vi "main.vi"(8 "error in":errorcluster) -> (0 "error out":errorcluster)   [LabVIEW 2018, in "Controller.lvlib"]
uses:
  Controller.lvlib
  Common/Common.lvlib
  Common/vi/Stop All - Action.ctl
  ctl/Queue Actions.ctl
  ctl/Module State.ctl
  Error Handler/Error Handler/ctl/Module State.ctl
  Error Handler/Error Handler/Error Handler.lvlib
  Entry Console/Entry Console.lvlib
  Wash Display Console/Wash Display Console.lvlib
  Vehicle Position Interface/Vehicle Position Interface.lvlib
  Vehicle Position Interface/ctl/Module State.ctl
  Wash Display Console/ctl/Module State.ctl
  Entry Console/ctl/Module State.ctl
  ctl/Database Action.ctl
  Entry Console/ctl/Wash Step Selection Buttons.ctl
  Common/ctl/Wash Step.ctl
  Common/ctl/Station.ctl
  ctl/Database Record.ctl
  ctl/Countdown Timer Action.ctl
  Vehicle Position Interface/ctl/Vehicle Position.ctl
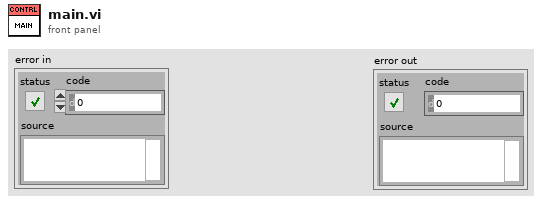
[diagram p1: front panel]
types:
  T1 = typedef "Entry Console.lvlib/Wash Step Selection Buttons.ctl" = cluster{"Under Body Wash":bool, "Bug Remover":bool, "Pre-Soak":bool, "High Pressure Wash (default)":bool, "Low Pressure Wax":bool, "Spot Free Rinse":bool, "Tire Shine Foam":bool, "Air Dry":bool}
  T2 = typedef "Common.lvlib/Wash Step.ctl" = enum16{"None", "Under Body Wash", "Bug Remover", "Pre-Soak", "High Pressure Wash (default)", "Low Pressure Wax", "Spot Free Rinse", "Tire Shine Foam", "Air Dry"}
  T3 = cluster{"Wash Steps Selected":T1, "Current Wash Step":T2, "Current State":enum16{"Wait", "Start", "Wait for vehicle Position", "Wash Step Execution", "Wash step/cycle completion", "Wash Step exit"}}
  T4 = typedef "Controller.lvlib/Module State.ctl" = enum16{"Init", "Idle", "Error", "Close", "Wait for Start State", "Start State", "Wait For Vehicle Position", "Wash Step Execution", "Wash Step/Cycle Completion", "Wash Exit State", "Wash Abort/Terminate State", "Entry Console: Start button pressed", "Entry Console: Wash Steps buttons Pressed", "Vehicle Position: Slider Moved", "Check Timer"}
  T5 = typedef "Controller.lvlib/Queue Actions.ctl" = enum16{"Create", "Get", "Destroy"}
  T6 = typedef "Common.lvlib/Stop All - Action.ctl" = enum16{"Create", "Get", "Fire", "Destroy"}
  T7 = typedef "Entry Console.lvlib/Module State.ctl" = enum16{"Init", "Idle", "Error", "Close", "Wash Step Selection Buttons: Enable/Disable All", "Wash Step Selection Buttons: Set All", "Wash Step Selection Buttons: Set Single (On/Off)", "Start: Enable/Disable", "Start: Set State (On/Off)"}
  T8 = typedef "Wash Display Console.lvlib/Module State.ctl" = enum16{"Init", "Idle", "Error", "Close", "Car Wash Indicators: Set All", "Car Wash Indicators: Set Single (On/Off)", "Wash Entry: Set State", "Vehicle Out of Position: Green/Red", "Time Remaining: Set"}
  T9 = typedef "Vehicle Position Interface.lvlib/Module State.ctl" = enum16{"Init", "Idle", "Error", "Close", "Vehicle Position: Set", "Vehicle Position: Send to controller"}
  T10 = typedef "Controller.lvlib/Database Action.ctl" = enum16{"Read Records (init)", "Get", "Query Timing Data", "Insert New Data record", "Update Data Record"}
  T11 = typedef "Error Handler.lvlib/Module State.ctl" = enum16{"Init", "Idle", "Error", "Close", "Handle External Error", "Log Error"}
  T12 = typedef "Controller.lvlib/Countdown Timer Action.ctl" = enum16{"Create (set goal time and start)", "Get (read)", "Reset"}
  T13 = typedef "Controller.lvlib/Database Record.ctl" = cluster{"Wash Step":T2, "Station":T14, "Wash Duration":dbl}
  T14 = typedef "Common.lvlib/Station.ctl" = enum16{"Entry", "Station 1", "Station 2", "Station 3", "Exit"}
  T15 = enum16{"Wait", "Start", "Wait for vehicle Position", "Wash Step Execution", "Wash step/cycle completion", "Wash Step exit"}
  T16 = typedef "Vehicle Position Interface.lvlib/Vehicle Position.ctl" = dbl
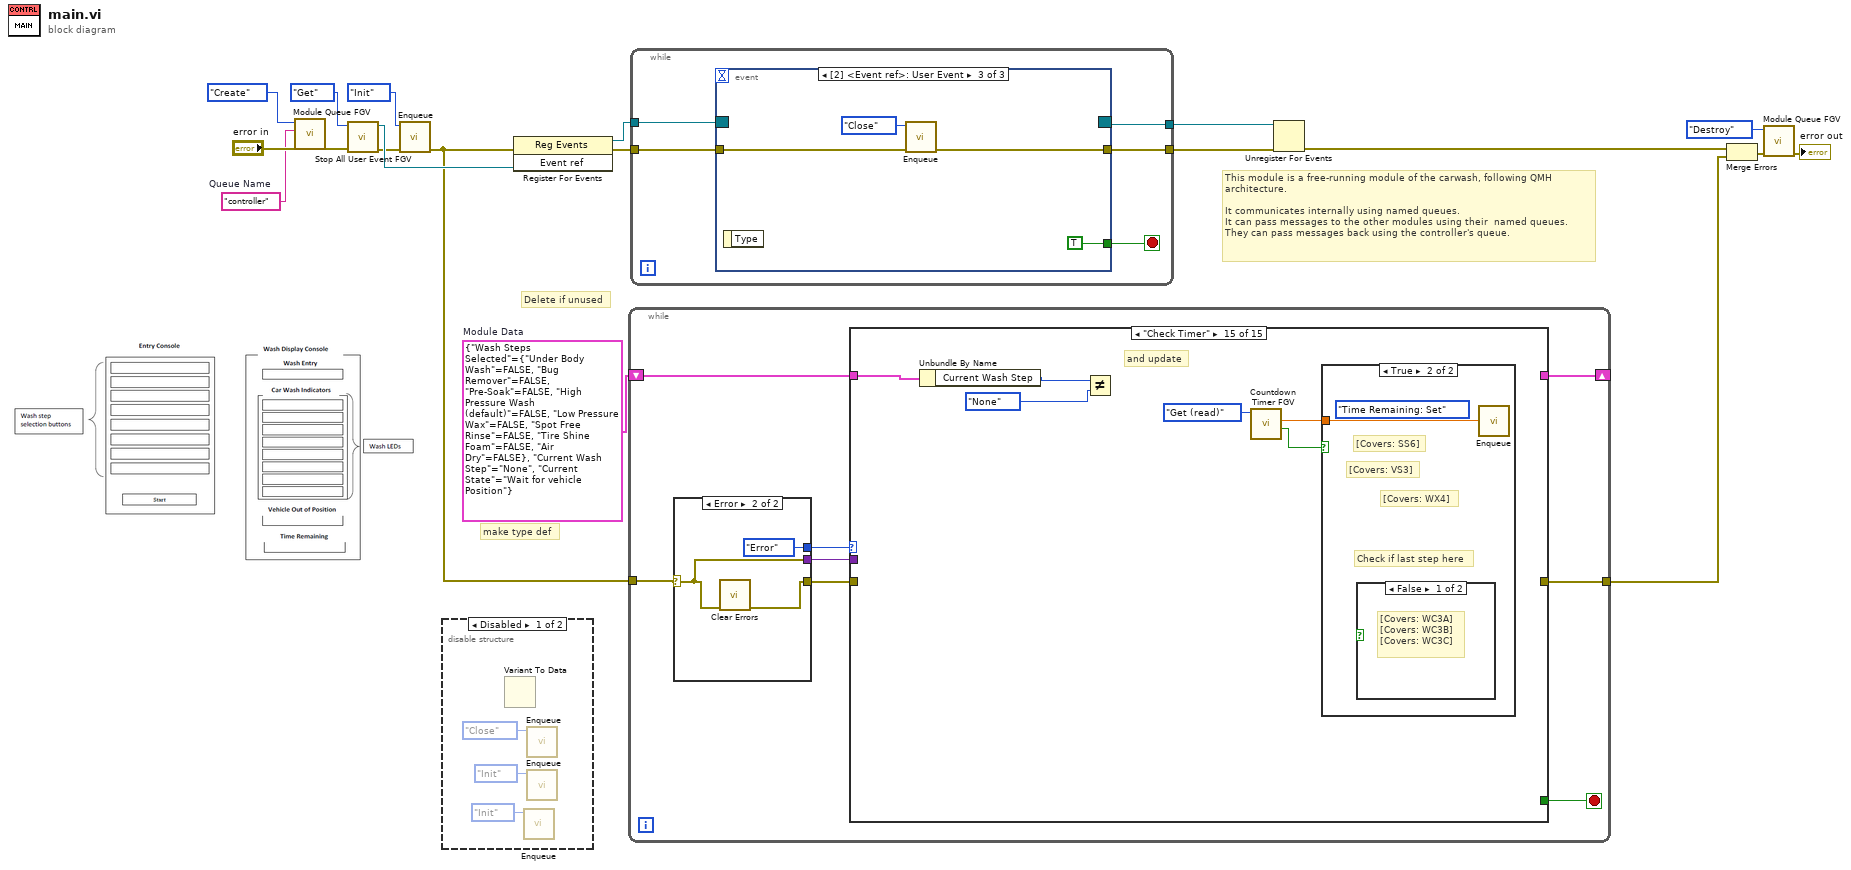
[diagram p0: block diagram]
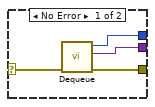
[diagram p3: hidden frame]
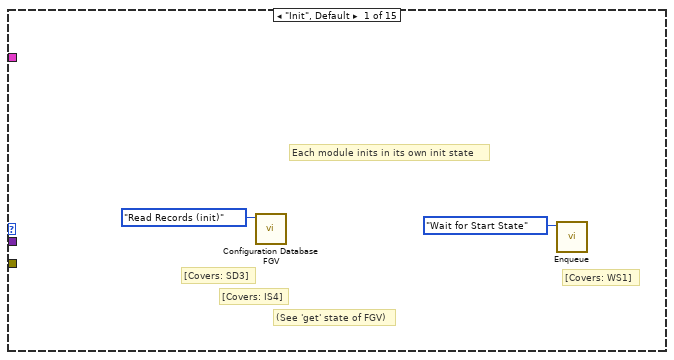
[diagram p4: hidden frame]
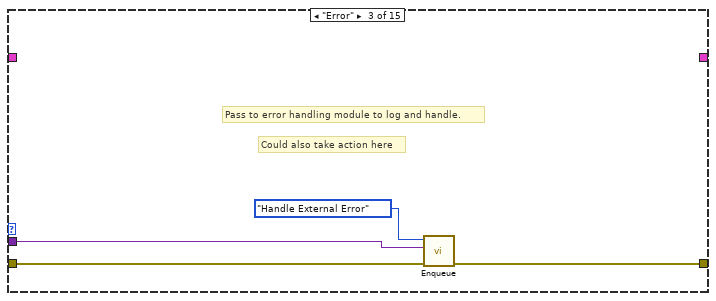
[diagram p6: hidden frame]
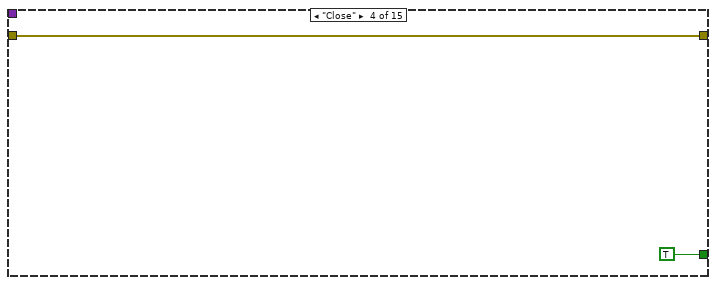
[diagram p7: hidden frame]
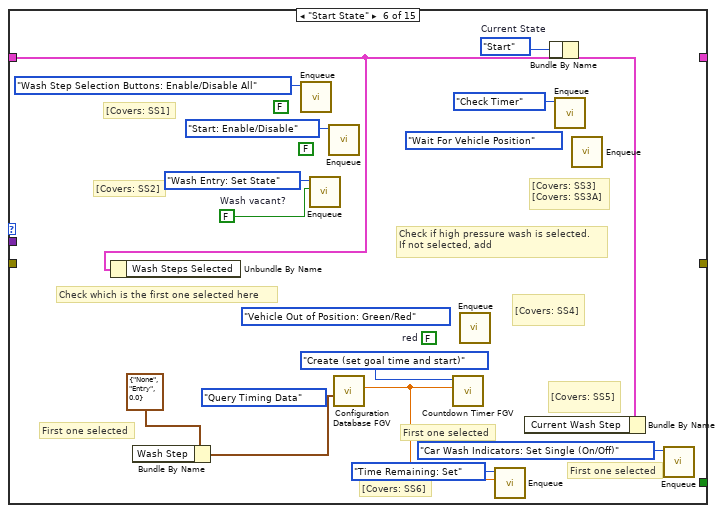
[diagram p9: hidden frame]
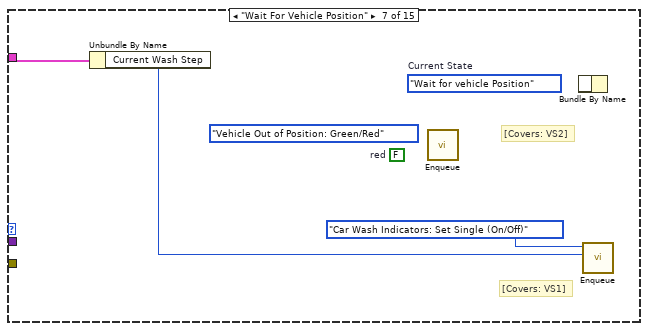
[diagram p10: hidden frame]
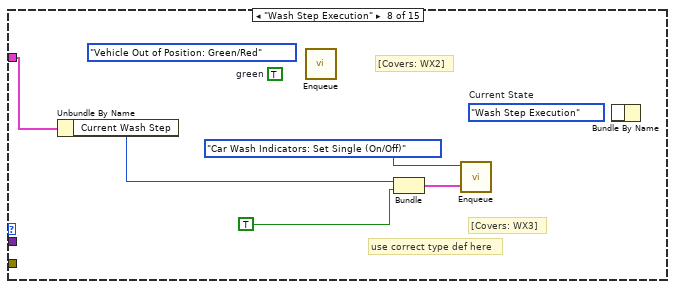
[diagram p11: hidden frame]
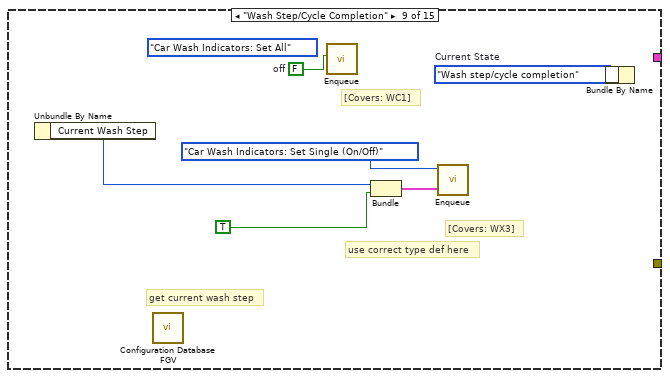
[diagram p12: hidden frame]
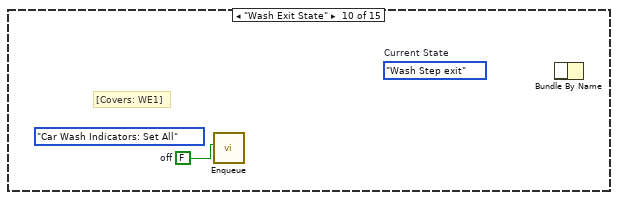
[diagram p13: hidden frame]
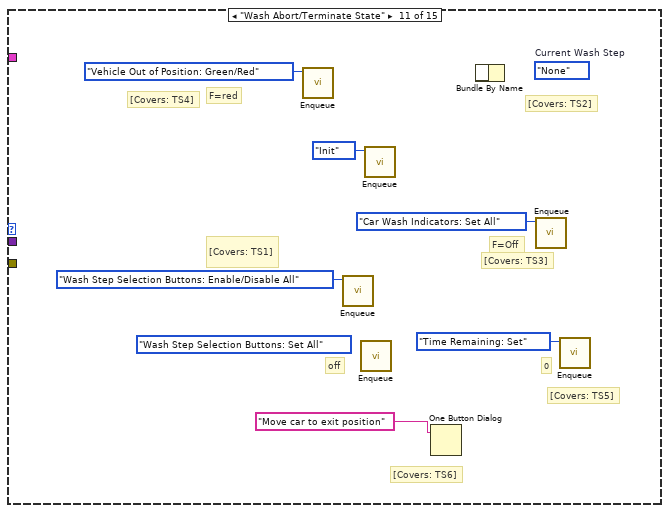
[diagram p14: hidden frame]
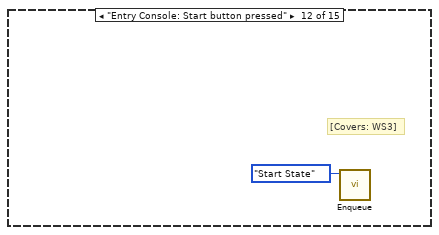
[diagram p15: hidden frame]
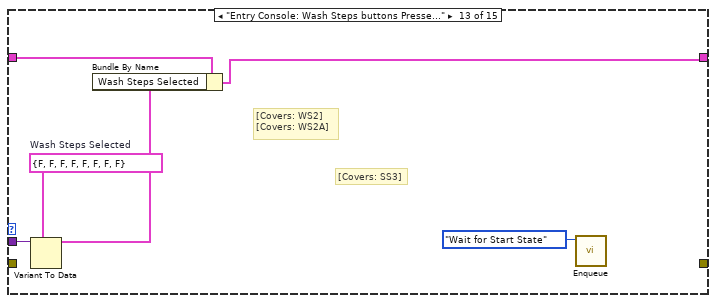
[diagram p16: hidden frame]
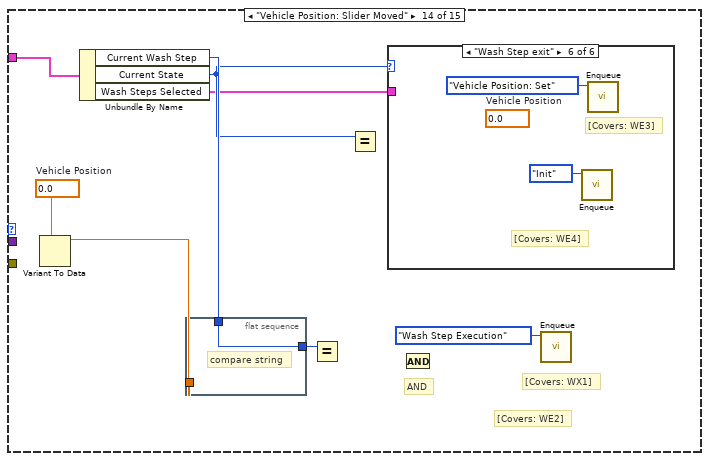
[diagram p17: hidden frame]
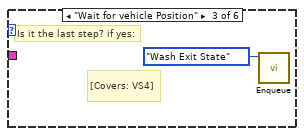
[diagram p20: hidden frame]
diagram:
  w1 = "controller"  # Queue Name
  w6 = T3 {"Wash Steps Selected"={"Under Body Wash"=FALSE, "Bug Remover"=FALSE, "Pre-Soak"=FALSE, "High Pressure Wash (default)"=FALSE, "Low Pressure Wax"=FALSE, "Spot Free Rinse"=FALSE, "Tire Shine Foam"=FALSE, "Air Dry"=FALSE}, "Current Wash Step"=enum."None", "Current State"=enum."Wait for vehicle Position"}  # Module Data
  # "make type def"
  # "This module is a free-running module of the carwash, following QMH\narchitecture.\n\nIt communicates internally using named queues.\nIt can pass messages to the other modules using their  named queues.\nThey can pass messages back using the controller's queue."
  # "Delete if unused"
  n1 = call "Module Queue FGV.vi"("error in"="error in", "Queue Name"=w1, "Action"=Queue_Actions."Create") -> ("error out"=w16:errorcluster)  [unwired: 7 in, 1 out]
  n2 = call "Stop All User Event FGV.vi"("error in"=w16, "Action"=Stop_All_-_Action."Get") -> ("error out"=w15:errorcluster, "Event ref"=w18:refnum<user-event>)  [unwired: 8 in]
  n3 = call "Enqueue.vi"("error in"=w15, "State"=Module_State."Init") -> ("error out"=w7:errorcluster)  [unwired: 9 in]
  n4 = disable-structure shown="Disabled" {
    frame Disabled {
      n5 = Variant To Data() -> ()  [unwired: 3 in, 2 out]
      n6 = call "Enqueue.vi"("State"=Module_State."Init") -> ()  [unwired: 10 in, 1 out]
      n7 = call "Enqueue.vi"("State"=Module_State."Close") -> ()  [unwired: 10 in, 1 out]
      n8 = call "Enqueue.vi"("State"=Module_State."Init") -> ()  [unwired: 10 in, 1 out]
    }
    frame Enabled {
    }
  }
  n9 = register-events(error in=w7, w18) -> (reference out=w13:refnum<event-registration>, error out=w11:errorcluster)  [unwired: 1 in]
  n10 = while {
    tunnel: w7 -> [w30]
    shift-right: [w25] -> _
    shift-left: w6 -> [w26]
    tunnel: [w23] -> w5
    stop <- w24 stop-if-true
    n11 = case shown="Error" w30 {
      selector: w30 -> [w34 w36]
      tunnel: [w33 w37] -> w27
      tunnel: [w32 w36] -> w28
      tunnel: [w31 Module_State."Error" ("State")] -> w29
      frame No Error {
        n12 = call "Dequeue.vi"("error in"=w34) -> ("error out"=w33:errorcluster, "Data"=w32:variant, "State"=w31:T4)  [unwired: 8 in]
      }
      frame Error {
        n13 = call <vilib>:"Clear Errors.vi"("error in (no error)"=w36) -> ("error out"=w37:errorcluster)  [unwired: 5 in, 1 out]
      }
    }
    n14 = case shown="\"Check Timer\"" w29 {
      tunnel: w28 -> [_ _ w42 _ _ _ _ _ _ _ _ _ w84 _ _]
      tunnel: w27 -> [_ _ w41 w45 _ _ _ _ _ _ _ _ _ _ _]
      tunnel: w26 -> [_ w40 _ _ _ w51 w63 w67 _ _ _ _ w86 w95 w104]
      tunnel: [_ w40 _ _ _ _ _ _ _ _ _ _ w82 _ _] -> w25
      tunnel: [_ _ _ TRUE _ _ _ _ _ _ _ _ _ _ _] -> w24
      tunnel: [_ _ w43 w45 _ _ _ _ _ _ _ _ _ _ _] -> w23
      frame "Init", Default {
        # "[Covers: WS1]"
        # "(See 'get' state of FGV)"
        # "[Covers: IS4]"
        # "Each module inits in its own init state"
        # "[Covers: SD3]"
        n15 = call "Configuration Database FGV.vi"("Action"=Database_Action."Read Records (init)") -> ()  [unwired: 8 in, 3 out]
        n16 = call "Enqueue.vi"("State"=Module_State."Wait for Start State") -> ()  [unwired: 10 in, 1 out]
      }
      frame "Idle" {
      }
      frame "Error" {
        # "Could also take action here"
        # "Pass to error handling module to log and handle."
        n17 = call "Enqueue.vi"("error in"=w41, "Data"=w42, "State"=Module_State."Handle External Error") -> ("error out"=w43:errorcluster)  [unwired: 8 in]
      }
      frame "Close" {
      }
      frame "Wait for Start State" {
        # "[Covers: WS1]"
      }
      frame "Start State" {
        w47 = T15."Start"  # Current State
        (unwired) Module_State."Wait For Vehicle Position" ("State")
        (unwired) FALSE  # red
        (unwired) Module_State."Vehicle Out of Position: Green/Red" ("State")
        w52 = FALSE  # Wash vacant?
        (unwired) FALSE
        (unwired) FALSE
        # "First one selected"
        # "Check which is the first one selected here"
        # "[Covers: SS5]"
        # "[Covers: SS6]"
        # "First one selected"
        # "[Covers: SS4]"
        # "[Covers: SS3]\n[Covers: SS3A]"
        # "[Covers: SS2]"
        # "[Covers: SS1]"
        # "First one selected"
        # "Check if high pressure wash is selected.\nIf not selected, add"
        n18 = Unbundle By Name(w51) -> ()  [unwired: 1 out]
        n19 = Bundle By Name(cluster=T13 {"Wash Step"=enum."None", "Station"=enum."Entry", "Wash Duration"=0.0} ("Record to add/replace/query")) -> (w56:T13)  [unwired: 1 in]
        n20 = call "Enqueue.vi"("State"=Module_State."Wash Step Selection Buttons: Enable/Disable All") -> ()  [unwired: 10 in, 1 out]
        n21 = call "Enqueue.vi"("Data"=w52, "State"=Module_State."Wash Entry: Set State") -> ()  [unwired: 9 in, 1 out]
        n22 = call "Enqueue.vi"("State"=Module_State."Start: Enable/Disable") -> ()  [unwired: 10 in, 1 out]
        n23 = call "Configuration Database FGV.vi"("Record to add/replace/query"=w56, "Action"=Database_Action."Query Timing Data") -> ("Wash Duration"=w50:dbl)  [unwired: 7 in, 2 out]
        n24 = call "Countdown Timer FGV.vi"("Goal time"=w50, "Action"=Countdown_Timer_Action."Create (set goal time and start)") -> ()  [unwired: 7 in, 3 out]
        n25 = call "Enqueue.vi"() -> ()  [unwired: 11 in, 1 out]
        n26 = call "Enqueue.vi"("Data"=w50, "State"=Module_State."Time Remaining: Set") -> ()  [unwired: 9 in, 1 out]
        n27 = Bundle By Name(cluster=w51) -> ()  [unwired: 1 in, 1 out]
        n28 = Bundle By Name(w47) -> ()  [unwired: 1 in, 1 out]
        n29 = call "Enqueue.vi"("State"=Module_State."Check Timer") -> ()  [unwired: 10 in, 1 out]
        n30 = call "Enqueue.vi"() -> ()  [unwired: 11 in, 1 out]
        n31 = call "Enqueue.vi"("State"=Module_State."Car Wash Indicators: Set Single (On/Off)") -> ()  [unwired: 10 in, 1 out]
      }
      frame "Wait For Vehicle Position" {
        (unwired) T15."Wait for vehicle Position"  # Current State
        (unwired) FALSE  # red
        (unwired) Module_State."Vehicle Out of Position: Green/Red" ("State")
        # "[Covers: VS2]"
        # "[Covers: VS1]"
        n32 = Unbundle By Name(w63) -> ("Current Wash Step"=w61:T2)
        n33 = call "Enqueue.vi"() -> ()  [unwired: 11 in, 1 out]
        n34 = Bundle By Name() -> ()  [unwired: 2 in, 1 out]
        n35 = call "Enqueue.vi"("Data"=w61, "State"=Module_State."Car Wash Indicators: Set Single (On/Off)") -> ()  [unwired: 9 in, 1 out]
      }
      frame "Wash Step Execution" {
        (unwired) T15."Wash Step Execution"  # Current State
        (unwired) TRUE  # green
        (unwired) Module_State."Vehicle Out of Position: Green/Red" ("State")
        # "use correct type def here"
        # "[Covers: WX3]"
        # "[Covers: WX2]"
        n36 = Unbundle By Name(w67) -> ("Current Wash Step"=w64:T2)
        n37 = call "Enqueue.vi"() -> ()  [unwired: 11 in, 1 out]
        n38 = Bundle("Current Wash Step"=w64, TRUE) -> (w66:cluster{"Current Wash Step":T2, bool})  [unwired: 1 in]
        n39 = call "Enqueue.vi"("Data"=w66, "State"=Module_State."Car Wash Indicators: Set Single (On/Off)") -> ()  [unwired: 9 in, 1 out]
        n40 = Bundle By Name() -> ()  [unwired: 2 in, 1 out]
      }
      frame "Wash Step/Cycle Completion" {
        w69 = FALSE  # off
        (unwired) Module_State."Car Wash Indicators: Set All" ("State")
        (unwired) T15."Wash step/cycle completion"  # Current State
        # "get current wash step"
        # "[Covers: WC1]"
        # "use correct type def here"
        # "[Covers: WX3]"
        n41 = Unbundle By Name() -> ("Current Wash Step"=w70:T2)  [unwired: 1 in]
        n42 = call "Configuration Database FGV.vi"() -> ()  [unwired: 9 in, 3 out]
        n43 = call "Enqueue.vi"("Data"=w69) -> ()  [unwired: 10 in, 1 out]
        n44 = Bundle("Current Wash Step"=w70, TRUE) -> (w72:cluster{"Current Wash Step":T2, bool})  [unwired: 1 in]
        n45 = call "Enqueue.vi"("Data"=w72, "State"=Module_State."Car Wash Indicators: Set Single (On/Off)") -> ()  [unwired: 9 in, 1 out]
        n46 = Bundle By Name() -> ()  [unwired: 2 in, 1 out]
      }
      frame "Wash Exit State" {
        w74 = FALSE  # off
        (unwired) Module_State."Car Wash Indicators: Set All" ("State")
        (unwired) T15."Wash Step exit"  # Current State
        # "[Covers: WE1]"
        n47 = call "Enqueue.vi"("Data"=w74) -> ()  [unwired: 10 in, 1 out]
        n48 = Bundle By Name() -> ()  [unwired: 2 in, 1 out]
      }
      frame "Wash Abort/Terminate State" {
        (unwired) Module_State."Wash Step Selection Buttons: Set All" ("State")
        (unwired) Wash_Step."None"  # Current Wash Step
        # "[Covers: TS5]"
        # "[Covers: TS6]"
        # "0"
        # "[Covers: TS3]"
        # "F=Off"
        # "[Covers: TS4]"
        # "F=red"
        # "off"
        # "[Covers: TS2]"
        # "[Covers: TS1]"
        n49 = call "Enqueue.vi"("State"=Module_State."Vehicle Out of Position: Green/Red") -> ()  [unwired: 10 in, 1 out]
        n50 = call "Enqueue.vi"("State"=Module_State."Wash Step Selection Buttons: Enable/Disable All") -> ()  [unwired: 10 in, 1 out]
        n51 = call "Enqueue.vi"() -> ()  [unwired: 11 in, 1 out]
        n52 = call "Enqueue.vi"("State"=Module_State."Init") -> ()  [unwired: 10 in, 1 out]
        n53 = One Button Dialog(message="Move car to exit position") -> ()  [unwired: 1 in, 1 out]
        n54 = Bundle By Name() -> ()  [unwired: 2 in, 1 out]
        n55 = call "Enqueue.vi"("State"=Module_State."Car Wash Indicators: Set All") -> ()  [unwired: 10 in, 1 out]
        n56 = call "Enqueue.vi"("State"=Module_State."Time Remaining: Set") -> ()  [unwired: 10 in, 1 out]
      }
      frame "Entry Console: Start button pressed" {
        # "[Covers: WS3]"
        n57 = call "Enqueue.vi"("State"=Module_State."Start State") -> ()  [unwired: 10 in, 1 out]
      }
      frame "Entry Console: Wash Steps buttons Pressed" {
        w83 = T1 {"Under Body Wash"=FALSE, "Bug Remover"=FALSE, "Pre-Soak"=FALSE, "High Pressure Wash (default)"=FALSE, "Low Pressure Wax"=FALSE, "Spot Free Rinse"=FALSE, "Tire Shine Foam"=FALSE, "Air Dry"=FALSE}  # Wash Steps Selected
        # "[Covers: SS3]"
        # "[Covers: WS2]\n[Covers: WS2A]"
        n58 = Variant To Data(type=w83, Variant=w84) -> (data=w85:T1)  [unwired: 1 in, 1 out]
        n59 = Bundle By Name(cluster=w86, "Wash Steps Selected"=w85) -> (w82:T3)
        n60 = call "Enqueue.vi"("State"=Module_State."Wait for Start State") -> ()  [unwired: 10 in, 1 out]
      }
      frame "Vehicle Position: Slider Moved" {
        w94 = T16 0.0 items=["Entry", "Station 1", "Station 2", "Station 3", "Exit"]  # Vehicle Position
        # "[Covers: WE2]"
        # "[Covers: WX1]"
        # "AND"
        n61 = Variant To Data(type=w94) -> (data=w92:T16)  [unwired: 2 in, 1 out]
        n62 = Unbundle By Name(w95) -> ("Current Wash Step"=w93:T2, "Current State"=w90:T15, "Wash Steps Selected"=w89:T1)
        n63 = flat-sequence {
          tunnel: w93 -> [w99]
          tunnel: w92 -> [_]
          tunnel: [w99] -> w88
          frame #0 {
            # "compare string"
          }
        }
        n64 = Equal?(x=w88) -> ()  [unwired: 1 in, 1 out]
        n65 = Equal?(x=w90) -> ()  [unwired: 1 in, 1 out]
        n66 = case shown="\"Wash Step exit\"" w90 {
          tunnel: w89 -> [_ _ _ _ _ _]
          frame "Wait", Default {
          }
          frame "Start" {
          }
          frame "Wait for vehicle Position" {
            # "[Covers: VS4]"
            # "Is it the last step? if yes:"
            n67 = call "Enqueue.vi"("State"=Module_State."Wash Exit State") -> ()  [unwired: 10 in, 1 out]
          }
          frame "Wash Step Execution" {
          }
          frame "Wash step/cycle completion" {
          }
          frame "Wash Step exit" {
            (unwired) T16 0.0 items=["Entry", "Station 1", "Station 2", "Station 3", "Exit"]  # Vehicle Position
            # "[Covers: WE4]"
            # "[Covers: WE3]"
            n68 = call "Enqueue.vi"("State"=Module_State."Init") -> ()  [unwired: 10 in, 1 out]
            n69 = call "Enqueue.vi"("State"=Module_State."Vehicle Position: Set") -> ()  [unwired: 10 in, 1 out]
          }
        }
        n70 = And() -> ()  [unwired: 2 in, 1 out]
        n71 = call "Enqueue.vi"("State"=Module_State."Wash Step Execution") -> ()  [unwired: 10 in, 1 out]
      }
      frame "Check Timer" {
        # "and update"
        n72 = Unbundle By Name(w104) -> ("Current Wash Step"=w102:T2)
        n73 = Not Equal?(x=w102, y=Wash_Step."None" ("Current Wash Step")) -> ()  [unwired: 1 out]
        n74 = call "Countdown Timer FGV.vi"("Action"=Countdown_Timer_Action."Get (read)") -> ("Time has elapsed?"=w101:bool, "Time remaining (s)"=w100:dbl)  [unwired: 8 in, 1 out]
        n75 = case shown="True" w101 {
          tunnel: w100 -> [_ w107]
          frame False {
            n76 = call "Enqueue.vi"("State"=Module_State."Check Timer") -> ()  [unwired: 10 in, 1 out]
          }
          frame True {
            (unwired) Module_State."Time Remaining: Set" ("State")
            # "Check if last step here"
            # "[Covers: WX4]"
            # "[Covers: VS3]"
            # "[Covers: SS6]"
            n77 = case shown="False" {
              selector: _ -> [_ _]
              frame False {
                # "[Covers: WC3A]\n[Covers: WC3B]\n[Covers: WC3C]"
              }
              frame True {
                # "[Covers: WC2A]\n[Covers: WC2B]\n[Covers: WC2C]"
              }
            }
            n78 = call "Enqueue.vi"("Data"=w107) -> ()  [unwired: 10 in, 1 out]
          }
        }
      }
    }
  }
  n79 = while {
    tunnel: w13 -> [w112]
    tunnel: [w111] -> w12
    tunnel: [w110] -> w10
    tunnel: w11 -> [w109]
    stop <- w108 stop-if-true
    n80 = event shown="[2] <Event ref>: User Event" {
      selector: w112 -> [_ _ _]
      dyn-events: [_ _ _] -> w111
      timeout: _ -> [_ _ _]
      tunnel: [w113 _ w116] -> w110
      tunnel: w109 -> [w113 _ w117]
      tunnel: [_ _ TRUE] -> w108
      event Timeout {
        n81 = event-data() -> ()  [unwired: 1 in, 1 out]
      }
      event Panel Close? {
        # "Seek further guidence."
        n82 = event-data() -> ()  [unwired: 1 in, 1 out]
        n83 = event-data() -> ()  [unwired: 2 in, 1 out]
      }
      event User Event {
        n84 = event-data() -> ()  [unwired: 1 in, 1 out]
        n85 = call "Enqueue.vi"("error in"=w117, "State"=Module_State."Close") -> ("error out"=w116:errorcluster)  [unwired: 9 in]
      }
    }
  }
  n86 = Unregister For Events(event registration refnum=w12, error in=w10) -> (error out=w2:errorcluster)
  n87 = Merge Errors(w2, w5) -> (w4:errorcluster)
  n88 = call "Module Queue FGV.vi"("error in"=w4, "Action"=Queue_Actions."Destroy") -> ("error out"=→"error out":errorcluster)  [unwired: 8 in, 1 out]
